vi "from string.vi"(8 "error in":errorcluster, 9 "data":string, 10 "version":string, 11 "configuration in":refnum<class "PL_Target Configuration.lvclass">) -> (0 "error out":errorcluster, 3 "configuration out":refnum<class "PL_Target Configuration.lvclass">)   [LabVIEW 2013, in "PL_Target Configuration.lvclass"]
doc: "Provides an interface for loading a module configuration from a file or other serialized data source. It is recommended that all children of this class store data in two sets--data required for its own initialization, and any data required for parent initialization--and that each implementation uses the <b>Call Parent Method</b> primitive to de-serialize parent information."
uses:
  PL_Target Configuration.lvclass
  <vilib>/NI/Tag Bus Module Framework/root configuration/Target Types.ctl
  PL_Target Configuration.lvclass/PL_Target Configuration.ctl
  <vilib>/NI/Tag Bus Module Framework/root configuration/TBM configuration.lvclass
  <vilib>/NI/Configuration Framework/serializable configuration/NISE_CEF_serializable configuration.lvclass
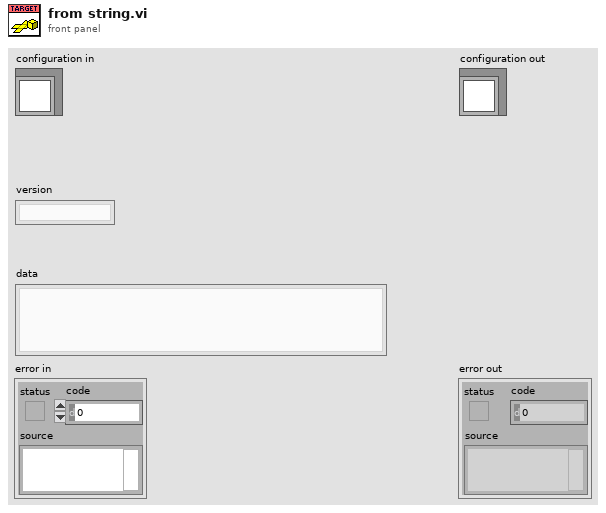
[diagram p1: front panel]
types:
  T1 = typedef "TBM configuration.lvclass/Target Types.ctl" = enum16{"Windows", "Mac", "Linux", "Linux RT ARM", "VxWorks", "Pharlap", "Other", "Linux RT x64"}
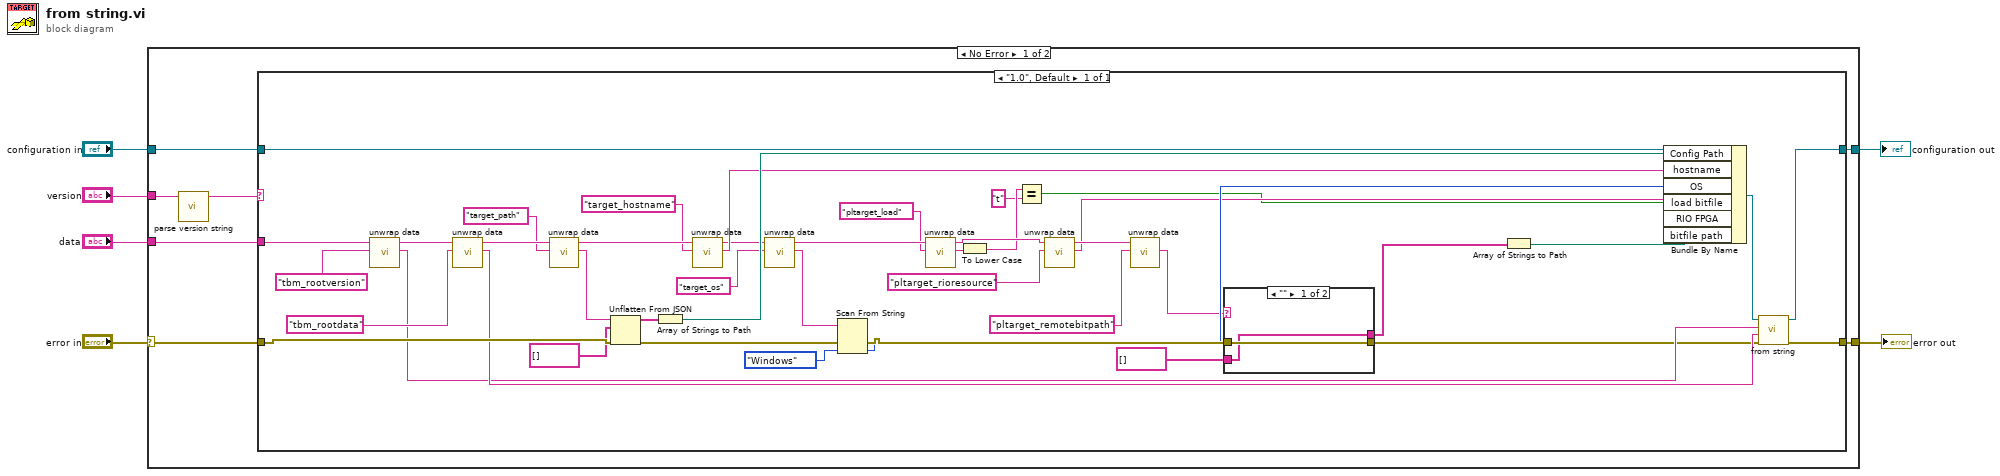
[diagram p0: block diagram]
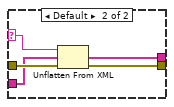
[diagram p2: hidden frame]
diagram:
  n1 = case shown="No Error" "error in" {
    selector: "error in" -> [w8 w65]
    tunnel: "data" -> [w13 _]
    tunnel: "configuration in" -> [w12 w64]
    tunnel: [w11 w64] -> w6
    tunnel: [w7 w65] -> w4
    tunnel: "version" -> [w10 _]
    frame No Error {
      n2 = call <vilib>:"parse version string.vi"("full version"=w10) -> ("major.minor version"=w9:string)  [unwired: 7 in, 3 out]
      n3 = case shown="\"1.0\", Default" w9 {
        tunnel: w13 -> [w54]
        tunnel: w8 -> [w55]
        tunnel: w12 -> [w56]
        tunnel: [w51] -> w11
        tunnel: [w53] -> w7
        frame "1.0", Default {
          n4 = call <vilib>:"unwrap data.vi"("identifier"="tbm_rootversion" ("additional identifier"), "data to unwrap"=w54) -> ("unwrapped data"=w38:string, "remaining string"=w42:string)  [unwired: 8 in]
          n5 = call <vilib>:"unwrap data.vi"("identifier"="tbm_rootdata" ("additional identifier"), "data to unwrap"=w42) -> ("unwrapped data"=w41:string, "remaining string"=w46:string)  [unwired: 8 in]
          n6 = call <vilib>:"unwrap data.vi"("identifier"="target_path" ("additional identifier"), "data to unwrap"=w46) -> ("unwrapped data"=w39:string, "remaining string"=w45:string)  [unwired: 8 in]
          n7 = Unflatten From JSON(JSON string=w39, type and defaults=string[] [] ("array of strings"), error in (no error)=w55) -> (value=w49:string[], error out=w50:errorcluster)  [unwired: 4 in]
          n8 = Array of Strings to Path(0:w49) -> (2:w47:path)  [unwired: 1 in]
          n9 = call <vilib>:"unwrap data.vi"("identifier"="target_hostname" ("additional identifier"), "data to unwrap"=w45) -> ("unwrapped data"=w36:string, "remaining string"=w35:string)  [unwired: 8 in]
          n10 = call <vilib>:"unwrap data.vi"("identifier"="target_os" ("additional identifier"), "data to unwrap"=w35) -> ("unwrapped data"=w32:string, "remaining string"=w27:string)  [unwired: 8 in]
          n11 = Scan From String(input string=w32, error in=w50, default 1=Target_Types."Windows" ("OS")) -> (error out=w33:errorcluster, output 1=w30:T1)  [unwired: 2 in, 2 out]
          n12 = call <vilib>:"unwrap data.vi"("identifier"="pltarget_load" ("additional identifier"), "data to unwrap"=w27) -> ("unwrapped data"=w25:string, "remaining string"=w28:string)  [unwired: 8 in]
          n13 = To Lower Case(string=w25) -> (all lower case string=w24:string)
          n14 = Equal?(x=w24, y="t") -> (x = y?=w22:bool)
          n15 = call <vilib>:"unwrap data.vi"("identifier"="pltarget_rioresource" ("additional identifier"), "data to unwrap"=w28) -> ("unwrapped data"=w26:string, "remaining string"=w29:string)  [unwired: 8 in]
          n16 = call <vilib>:"unwrap data.vi"("identifier"="pltarget_remotebitpath" ("additional identifier"), "data to unwrap"=w29) -> ("unwrapped data"=w17:string)  [unwired: 8 in, 1 out]
          n17 = case shown="\"\"" w17 {
            selector: w17 -> [_ w59]
            tunnel: w33 -> [w58 w63]
            tunnel: [w58 w62] -> w21
            tunnel: string[] [] ("array of strings") -> [w57 w61]
            tunnel: [w57 w60] -> w18
            frame "" {
            }
            frame Default {
              n18 = Unflatten From XML(xml string=w59, type=w61, error in (no error)=w63) -> (value=w60:string[], error out=w62:errorcluster)
            }
          }
          n19 = Array of Strings to Path(0:w18) -> (2:w20:path)  [unwired: 1 in]
          n20 = Bundle By Name(cluster=w56, "Config Path"=w47, "hostname"=w36, "OS"=w30, "load bitfile"=w22, "RIO FPGA"=w26, "bitfile path"=w20) -> (w52:refnum<class "PL_Target Configuration.lvclass">)
          n21 = call-parent "from string.vi"("error in"=w21, "data"=w41, "version"=w38, "configuration in"=w52) -> ("error out"=w53:errorcluster, "configuration out"=w51:refnum<class "PL_Target Configuration.lvclass">)  [unwired: 6 in]
        }
      }
    }
    frame Error {
    }
  }
  "error out" <- w4
  "configuration out" <- w6
